vi "Oscilloscope.vi"(0 "Trigger Source":u16(ring) caption="SCOPET_Source" items=["Immediate", "TRIGGER", "SYNC_OUT", "CH A", "CH B"], 1 "ChA_Source":u16, 2 "ChB_Source":u16, 3 "Device Name":tag="Dev1", 5 "Trigger Type":u16(ring) caption="SCOPET_Type" items=["Digital", "Analog"], 7 "Slope":i32(ring) caption="SCOPET_Slope" items=["Positive", "Negative"], 9 "Level":dbl caption="SCOPET_Level", 11 "Sample Rate (Hz)":dbl=100000.0 caption="SCOPEH_SampleRate" min=0.0 step=1000000.0 format="%#_4p", 12 "Record Length":i32=2000 caption="SCOPEH_RecordLength" min=5 max=75000000 step=1 format="%#.9p", 13 "Acquire":u16(ring)=10178 caption="SCOPEH_Acquire" items=["N Samples"=10178, "Continuously"=10123]) -> (4 "CH A":T1, 6 "CH B":T1, 8 "Record count":i32, 10 "Waveform Graph":dbl[][](graph), 15 "interleaved array":dbl[](array[numeric]))   [LabVIEW 2010]
uses:
  <vilib>/DAQmx/create/channels.llb/DAQmx Create Channel (AI-Voltage-Basic).vi
  <vilib>/DAQmx/configure/timing.llb/DAQmx Timing (Sample Clock).vi
  Program Files (x86)/National Instruments/LabVIEW 2011/resource/objmgr/daqmx.rc
  <vilib>/DAQmx/read.llb/DAQmx Read (Analog 2D DBL NChan NSamp).vi
  <vilib>/Analysis/Matrix/NI_Matrix.lvlib
  <vilib>/Analysis/Matrix/Numeric/Conversions/Array To Matrix - RA.vi
  <vilib>/Analysis/Matrix/Datatypes/RealMatrix.ctl
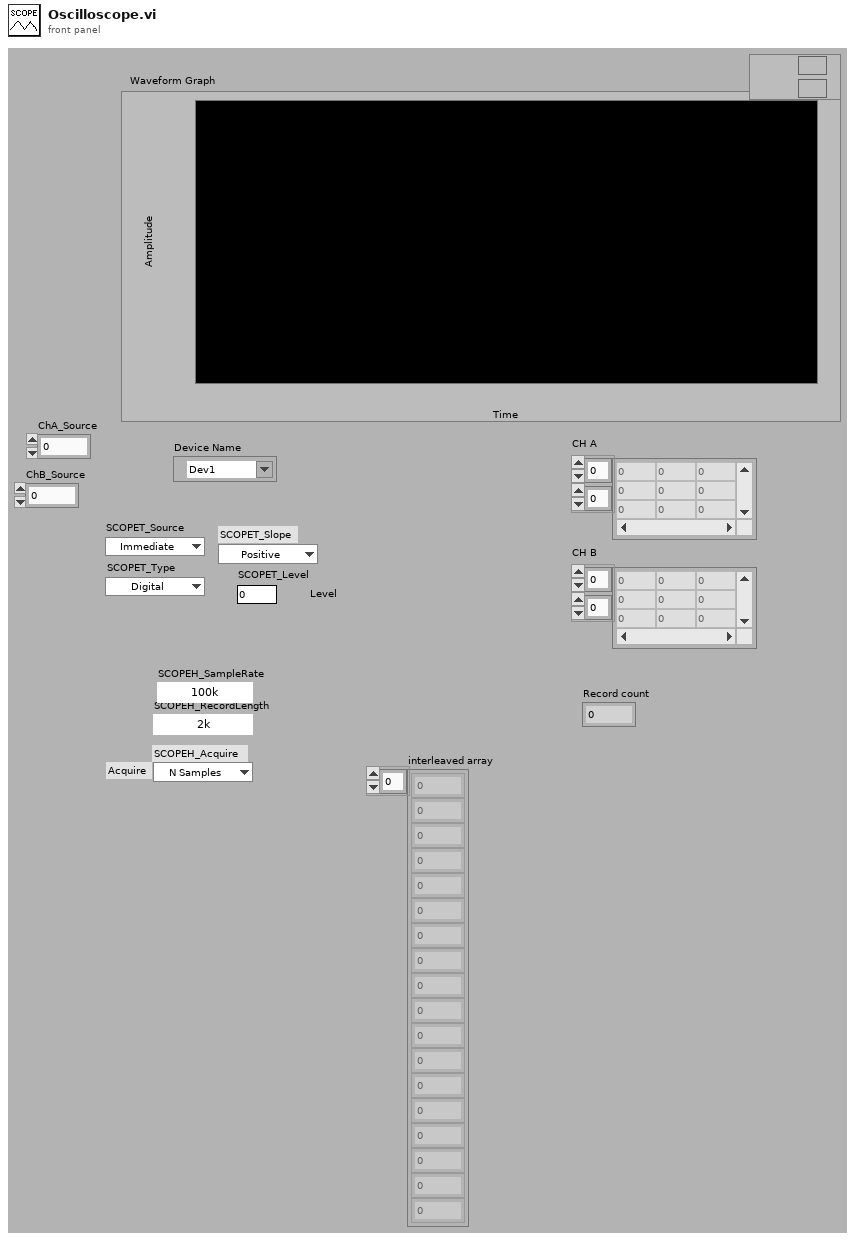
[diagram p1: front panel]
types:
  T1 = typedef "NI_Matrix.lvlib/RealMatrix.ctl" = dbl[][]
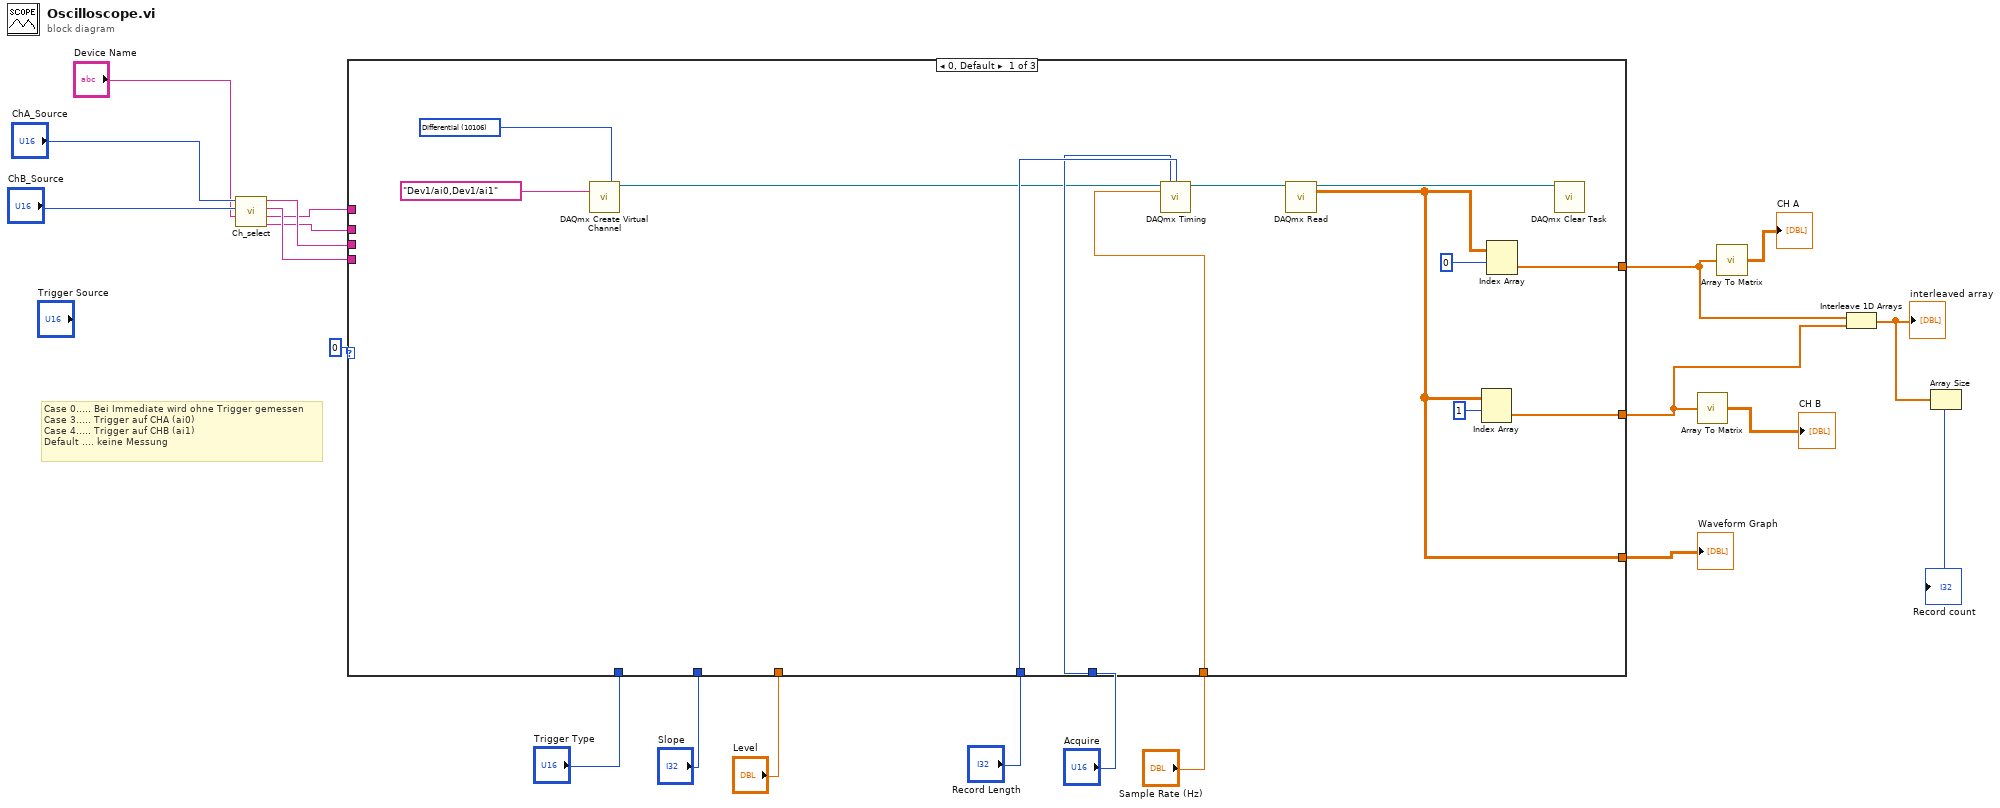
[diagram p0: block diagram]
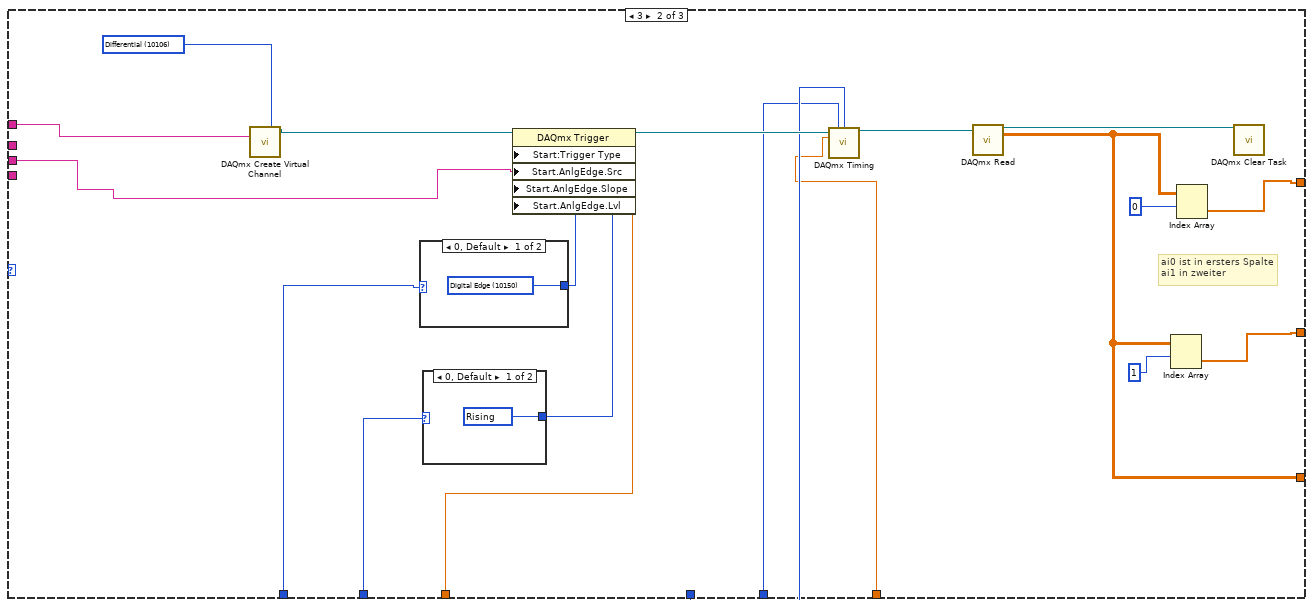
[diagram p2: hidden frame]
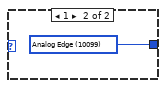
[diagram p3: hidden frame]
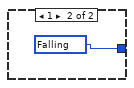
[diagram p4: hidden frame]
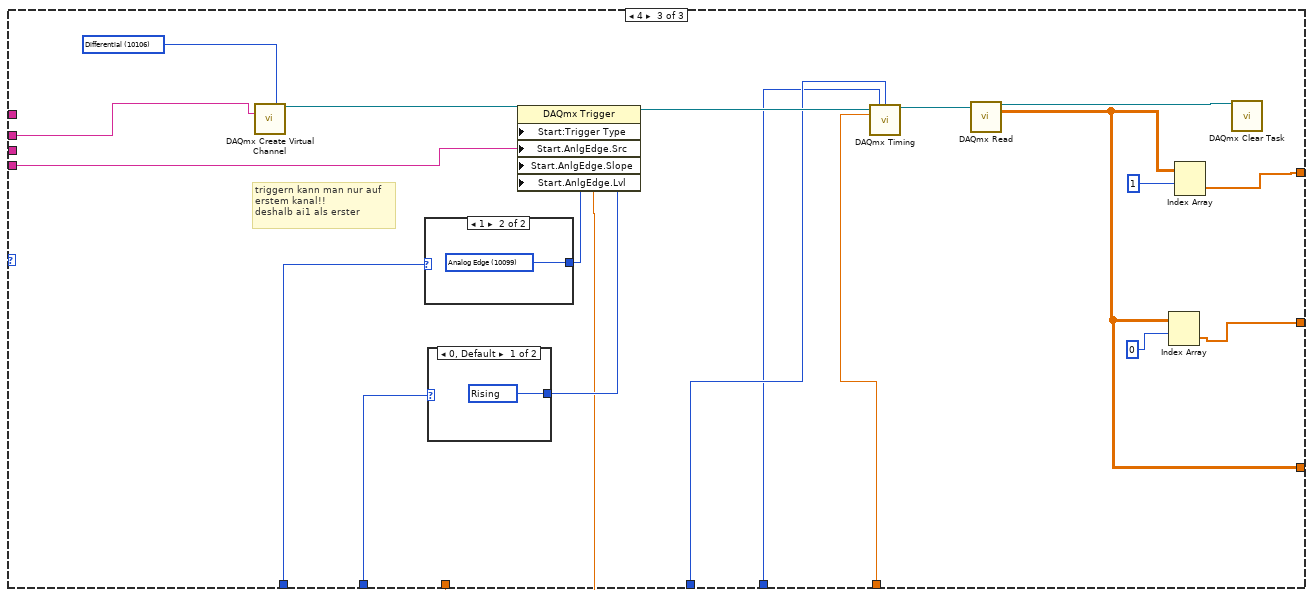
[diagram p5: hidden frame]
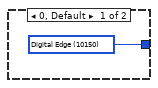
[diagram p6: hidden frame]
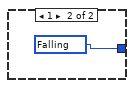
[diagram p7: hidden frame]
diagram:
  # "Case 0..... Bei Immediate wird ohne Trigger gemessen\nCase 3..... Trigger auf CHA (ai0)\nCase 4..... Trigger auf CHB (ai1)\nDefault .... keine Messung"
  n1 = call "Ch_select.vi"("Device Name"="Device Name", "ChB_Source"="ChB_Source", "ChA_Source"="ChA_Source") -> ("CHBA"=w5:tag, "CHAB"=w6:tag, "CHB"=w7:tag, "CHA"=w8:tag)  [unwired: 3 in]
  n2 = case shown="0, Default" u16 0 ("Trigger Source") {
    tunnel: "Trigger Type" -> [_ w47 w69]
    tunnel: "Slope" -> [_ w46 w68]
    tunnel: "Level" -> [_ w45 w67]
    tunnel: "Record Length" -> [w29 w43 w66]
    tunnel: "Acquire" -> [w28 w42 w65]
    tunnel: [w26 w39 w63] -> w14
    tunnel: [w25 w40 w64] -> w13
    tunnel: [w24 w41 w62] -> w12
    tunnel: w6 -> [_ w38 _]
    tunnel: w8 -> [_ w37 _]
    tunnel: w5 -> [_ _ w61]
    tunnel: "Sample Rate (Hz)" -> [w23 w35 w60]
    tunnel: w7 -> [_ _ w59]
    frame 0, Default {
      w31 = 10106 items=["default"=-1, "RSE"=10083, "NRSE"=10078, "Differential"=10106, "Pseudodifferential"=12529] ("input terminal configuration")
      n3 = call-poly <vilib>:"DAQmx Create Virtual Channel.vi"("input terminal configuration"=w31, "physical channels"=tag "Dev1/ai0,Dev1/ai1") -> ("task out"=w27:refnum<k21>)  [unwired: 12 in, 1 out]
      n4 = call-poly <vilib>:"DAQmx Timing.vi"("task/channels in"=w27, "sample mode"=w28, "samples per channel"=w29, "rate"=w23) -> ("task out"=w30:refnum<k21>)  [unwired: 10 in, 1 out]
      n5 = call-poly <vilib>:"DAQmx Read.vi"("task/channels in"=w30) -> ("task out"=w34:refnum<k21>, "data"=w24:dbl[][])  [unwired: 12 in, 1 out]
      n6 = Index Array(array=w24, index (row)=1) -> (element=w25:dbl[])  [unwired: 1 in]
      n7 = Index Array(array=w24, index (row)=0) -> (element=w26:dbl[])  [unwired: 1 in]
      n8 = call <vilib>:"DAQmx Clear Task.vi"("task in"=w34) -> ()  [unwired: 14 in, 1 out]
    }
    frame 3 {
      w53 = 10106 items=["default"=-1, "RSE"=10083, "NRSE"=10078, "Differential"=10106, "Pseudodifferential"=12529] ("input terminal configuration")
      # "ai0 ist in ersters Spalte\nai1 in zweiter"
      n9 = call-poly <vilib>:"DAQmx Create Virtual Channel.vi"("input terminal configuration"=w53, "physical channels"=w38) -> ("task out"=w36:refnum<k21>)  [unwired: 12 in, 1 out]
      n10 = case shown="0, Default" w47 {
        tunnel: [w55 w56] -> w49
        frame 0, Default {
          w55 = 10150 items=["Analog Edge"=10099, "Digital Edge"=10150, "Digital Pattern"=10398, "Analog Window"=10103, "None"=10230] ("Start.TrigType")
        }
        frame 1 {
          w56 = 10099 items=["Analog Edge"=10099, "Digital Edge"=10150, "Digital Pattern"=10398, "Analog Window"=10103, "None"=10230] ("Start.TrigType")
        }
      }
      n11 = case shown="0, Default" w46 {
        tunnel: [w57 w58] -> w48
        frame 0, Default {
          w57 = 10280 items=["Rising"=10280, "Falling"=10171] ("Start.DigEdge.Edge")
        }
        frame 1 {
          w58 = 10171 items=["Rising"=10280, "Falling"=10171] ("Start.DigEdge.Edge")
        }
      }
      n12 = property class="DAQmx Trigger"(reference=w36, "Start:Trigger Type"=w49, "Start.AnlgEdge.Src"=w37, "Start.AnlgEdge.Slope"=w48, "Start.AnlgEdge.Lvl"=w45) -> (reference out=w44:refnum<k21>)  [unwired: 1 in, 1 out]
      n13 = call-poly <vilib>:"DAQmx Timing.vi"("task/channels in"=w44, "sample mode"=w42, "samples per channel"=w43, "rate"=w35) -> ("task out"=w54:refnum<k21>)  [unwired: 10 in, 1 out]
      n14 = call-poly <vilib>:"DAQmx Read.vi"("task/channels in"=w54) -> ("task out"=w50:refnum<k21>, "data"=w41:dbl[][])  [unwired: 12 in, 1 out]
      n15 = Index Array(array=w41, index (row)=1) -> (element=w40:dbl[])  [unwired: 1 in]
      n16 = Index Array(array=w41, index (row)=0) -> (element=w39:dbl[])  [unwired: 1 in]
      n17 = call <vilib>:"DAQmx Clear Task.vi"("task in"=w50) -> ()  [unwired: 14 in, 1 out]
    }
    frame 4 {
      w71 = 10106 items=["default"=-1, "RSE"=10083, "NRSE"=10078, "Differential"=10106, "Pseudodifferential"=12529] ("input terminal configuration")
      # "triggern kann man nur auf\nerstem kanal!!\ndeshalb ai1 als erster"
      n18 = call-poly <vilib>:"DAQmx Create Virtual Channel.vi"("input terminal configuration"=w71, "physical channels"=w61) -> ("task out"=w77:refnum<k21>)  [unwired: 12 in, 1 out]
      n19 = case shown="1" w69 {
        tunnel: [w79 w80] -> w75
        frame 0, Default {
          w79 = 10150 items=["Analog Edge"=10099, "Digital Edge"=10150, "Digital Pattern"=10398, "Analog Window"=10103, "None"=10230] ("Start.TrigType")
        }
        frame 1 {
          w80 = 10099 items=["Analog Edge"=10099, "Digital Edge"=10150, "Digital Pattern"=10398, "Analog Window"=10103, "None"=10230] ("Start.TrigType")
        }
      }
      n20 = case shown="0, Default" w68 {
        tunnel: [w81 w82] -> w76
        frame 0, Default {
          w81 = 10280 items=["Rising"=10280, "Falling"=10171] ("Start.DigEdge.Edge")
        }
        frame 1 {
          w82 = 10171 items=["Rising"=10280, "Falling"=10171] ("Start.DigEdge.Edge")
        }
      }
      n21 = property class="DAQmx Trigger"(reference=w77, "Start:Trigger Type"=w75, "Start.AnlgEdge.Src"=w59, "Start.AnlgEdge.Slope"=w76, "Start.AnlgEdge.Lvl"=w67) -> (reference out=w78:refnum<k21>)  [unwired: 1 in, 1 out]
      n22 = call-poly <vilib>:"DAQmx Timing.vi"("task/channels in"=w78, "sample mode"=w65, "samples per channel"=w66, "rate"=w60) -> ("task out"=w70:refnum<k21>)  [unwired: 10 in, 1 out]
      n23 = call-poly <vilib>:"DAQmx Read.vi"("task/channels in"=w70) -> ("task out"=w74:refnum<k21>, "data"=w62:dbl[][])  [unwired: 12 in, 1 out]
      n24 = Index Array(array=w62, index (row)=0) -> (element=w64:dbl[])  [unwired: 1 in]
      n25 = Index Array(array=w62, index (row)=1) -> (element=w63:dbl[])  [unwired: 1 in]
      n26 = call <vilib>:"DAQmx Clear Task.vi"("task in"=w74) -> ()  [unwired: 14 in, 1 out]
    }
  }
  "Waveform Graph" <- w12
  n27 = call-poly <vilib>:"Array To Matrix.vi"("Real 1D Array"=w13) -> ("Real Matrix (Column Vector)"=→"CH B":T1)
  n28 = call-poly <vilib>:"Array To Matrix.vi"("Real 1D Array"=w14) -> ("Real Matrix (Column Vector)"=→"CH A":T1)
  n29 = Interleave 1D Arrays(w14, w13) -> (w11:dbl[])
  "interleaved array" <- w11
  n30 = Array Size(array=w11) -> (size(s)=→"Record count":i32)
